vi "Apply Layouts To Objects.vi"(5 "scaling settings":T1={"scaling factor"={"horizontal"=1.0, "vertical"=1.0}, "scale text"=FALSE} {"scaling factor"."vertical" min=0.0; "scaling factor"."horizontal" min=0.0}, 7 "properties to ignore":variant, 8 "error in":errorcluster, 9 "GObj refnums":refnum<vi>[](array[refnum]), 10 "object ID list in":variant, 11 "object layouts in":refnum<class "Object Layout.lvclass">[](array[class])) -> (0 "error out":errorcluster, 2 "object ID list out":variant, 3 "object layouts out":refnum<class "Object Layout.lvclass">[](array[class]))   [LabVIEW 2010, in "NI_SE_Front Panel Layout.lvlib"]
uses:
  NI_SE_Front Panel Layout.lvlib
  Object Layout Classes/Object Layout/Object Layout.lvclass
  Scaling Factor_Options.ctl
  XY Scaling Factor.ctl
  Object Layout Classes/Object Layout/Object Layout.lvclass/Object Layout.ctl
  Object Layout Classes/Object Layout/Get Unique Name.vi
  Object Layout Classes/Object Layout/Get UID.vi
  Convert UID To String.vi
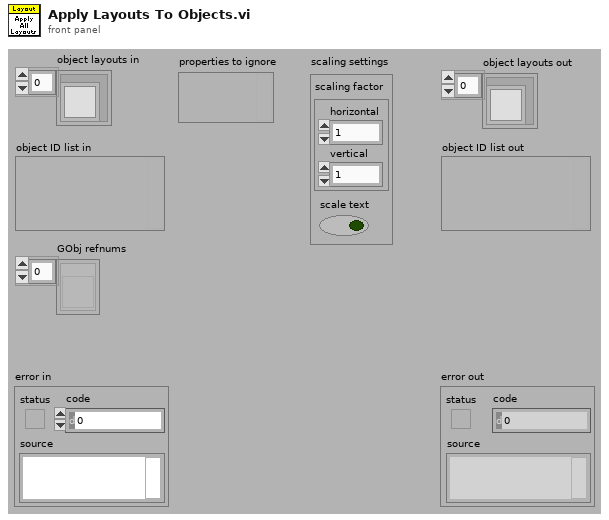
[diagram p1: front panel]
types:
  T1 = typedef "NI_SE_Front Panel Layout.lvlib/Scaling Factor_Options.ctl" = cluster{"scaling factor":T2, "scale text":bool}
  T2 = typedef "NI_SE_Front Panel Layout.lvlib/XY Scaling Factor.ctl" = cluster{"horizontal":dbl, "vertical":dbl}
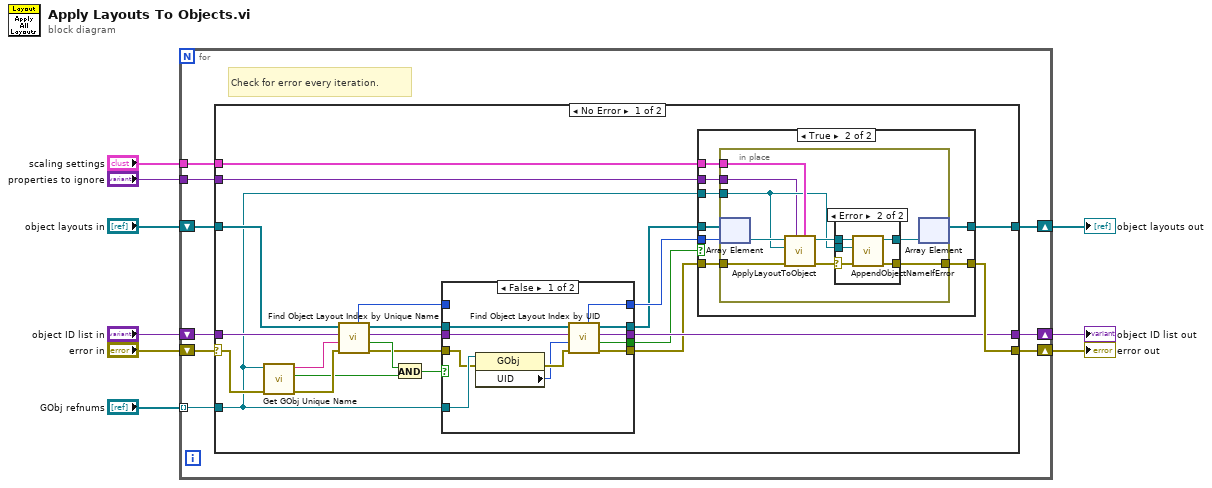
[diagram p0: block diagram]
diagram:
  n1 = for {
    tunnel: "GObj refnums" -> [w18] mode=indexing
    shift-right: [w16] -> w8
    shift-left: "error in" -> [w17]
    tunnel: "scaling settings" -> [w15]
    shift-right: [w11] -> w1
    shift-left: "object layouts in" -> [w14]
    shift-right: [w12] -> w6
    shift-left: "object ID list in" -> [w13]
    tunnel: "properties to ignore" -> [w10]
    # "Check for error every iteration."
    n2 = case shown="No Error" w17 {
      selector: w17 -> [w36 w85]
      tunnel: w18 -> [w28 _]
      tunnel: [w40 w85] -> w16
      tunnel: w15 -> [w39 _]
      tunnel: w14 -> [w35 w84]
      tunnel: w13 -> [w34 w83]
      tunnel: [w21 w83] -> w12
      tunnel: [w38 w84] -> w11
      tunnel: w10 -> [w37 _]
      frame No Error {
        n3 = call "Get GObj Unique Name.vi"("error in"=w36, "GObj Refnum"=w28) -> ("error out"=w32:errorcluster, "found?"=w31:bool, "unique name"=w33:string)  [unwired: 7 in]
        n4 = call "Find Object Layout Index by Unique Name.vi"("error in"=w32, "unique name"=w33, "object ID list in"=w34, "object layouts in"=w35) -> ("error out"=w27:errorcluster, "found?"=w30:bool, "object ID list out"=w25:variant, "object layouts out"=w26:refnum<class "Object Layout.lvclass">[], "object layout index"=w24:i32)  [unwired: 3 in]
        n5 = And(x=w30, y=w31) -> (x .and. y?=w29:bool)
        n6 = case shown="False" w29 {
          selector: w29 -> [_ w52]
          tunnel: w28 -> [w51 _]
          tunnel: w27 -> [w50 w53]
          tunnel: w26 -> [w49 w54]
          tunnel: w25 -> [w46 w55]
          tunnel: w24 -> [_ w56]
          tunnel: [w41 w56] -> w23
          tunnel: [w45 w55] -> w21
          tunnel: [w44 w54] -> w22
          tunnel: [w42 w53] -> w20
          tunnel: [w43 w52] -> w19
          frame False {
            n7 = property class="GObj"(reference=w51, error in=w50) -> (error out=w48:errorcluster, "UID"=w47:i32)  [unwired: 1 out]
            n8 = call "Find Object Layout Index by UID.vi"("error in (no error)"=w48, "unique name"=w47, "object ID list in"=w46, "object layouts in"=w49) -> ("error out"=w42:errorcluster, "found?"=w43:bool, "object ID list out"=w45:variant, "object layouts out"=w44:refnum<class "Object Layout.lvclass">[], "object layout index"=w41:i32)  [unwired: 3 in]
          }
          frame True {
          }
        }
        n9 = case shown="True" w19 {
          tunnel: w28 -> [_ w66]
          tunnel: [w57 w65] -> w40
          tunnel: w23 -> [_ w64]
          tunnel: [w58 w63] -> w38
          tunnel: w39 -> [_ w62]
          tunnel: w22 -> [w58 w61]
          tunnel: w20 -> [w57 w60]
          tunnel: w37 -> [_ w59]
          frame False {
          }
          frame True {
            n10 = in-place {
              in-place-border: w66 -> [w69]
              in-place-border: w60 -> [w75]
              in-place-border: [w70] -> w65
              in-place-border: w62 -> [w73]
              in-place-border: w59 -> [w67]
              n11 = in-place-array #1(w61, w64) -> (w74:refnum<class "Object Layout.lvclass">)
              n12 = call-dynamic "ApplyLayoutToObject.vi"("scaling settings"=w73, "properties to ignore"=w67, "error in (no error)"=w75, "GObj Refnum"=w69, "Object Layout in"=w74) -> ("error out"=w68:errorcluster, "Object Layout out"=w72:refnum<class "Object Layout.lvclass">)  [unwired: 5 in]
              n13 = case shown="Error" w68 {
                selector: w68 -> [w76 w78]
                tunnel: w72 -> [w77 w82]
                tunnel: [w77 w81] -> w71
                tunnel: [w76 w80] -> w70
                tunnel: w69 -> [_ w79]
                frame No Error {
                }
                frame Error {
                  n14 = call-dynamic "AppendObjectNameIfError.vi"("error in (no error)"=w78, "GObj Refnum"=w79, "Object Layout in"=w82) -> ("error out"=w80:errorcluster, "Object Layout out"=w81:refnum<class "Object Layout.lvclass">)  [unwired: 7 in]
                }
              }
              n15 = in-place-array #1(w71) -> (w63:refnum<class "Object Layout.lvclass">[])  [unwired: 1 out]
            }
          }
        }
      }
      frame Error {
      }
    }
  }
  "error out" <- w8
  "object ID list out" <- w6
  "object layouts out" <- w1
